vi "Enable Monitoring All Labels on Channel.vi"(8 "error in":errorcluster, 10 "channel number":u8, 11 "board handle":u8) -> (0 "error out":errorcluster, 2 "channel number out":u8, 3 "board handle out":u8)   [LabVIEW 2020, in "AIM ARINC 429 Hardware API.lvlib"]
uses:
  AIM ARINC 429 Hardware API.lvlib
  <instrlib>/AIM GmbH/_ARINC-429/subvi/Error Converter (ErrCode or Status).vi
  <instrlib>/AIM GmbH/_ARINC-429/subvi/Get Library Path.vi
  <instrlib>/AIM GmbH/_ARINC-429/VIs/Library/Api429Lib Error Desc Get.vi
  <instrlib>/AIM GmbH/_ARINC-429/subvi/Get Error Number Offset.vi
  <vilib>/Utility/error.llb/Error Cluster From Error Code.vi
  <instrlib>/AIM GmbH/_ARINC-429/AIM429LV.lvlib
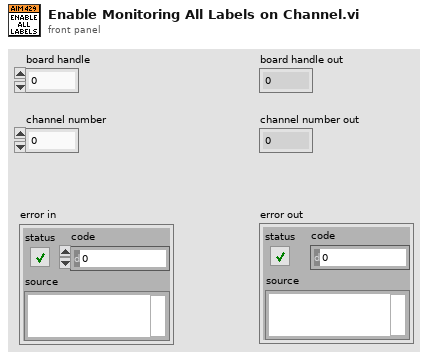
[diagram p1: front panel]
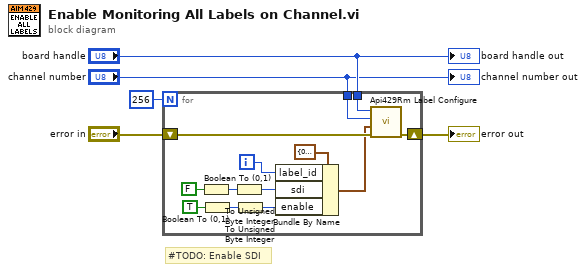
[diagram p0: block diagram]
diagram:
  # "#TODO: Enable SDI"
  n1 = for {
    N: 256 -> [_]
    tunnel: "board handle" -> [w18]
    tunnel: "channel number" -> [w17]
    shift-right: [w15] -> w2
    shift-left: "error in" -> [w16]
    i -> [w12]
    n2 = Boolean To (0,1)(Boolean=FALSE) -> (0, 1=w11:i16)
    n3 = Boolean To (0,1)(Boolean=TRUE) -> (0, 1=w7:i16)
    n4 = To Unsigned Byte Integer(number=w11) -> (unsigned 8bit integer=w9:u8)
    n5 = To Unsigned Byte Integer(number=w7) -> (unsigned 8bit integer=w6:u8)
    n6 = Bundle By Name(cluster=cluster{"label_id":u32, "sdi":u32, "enable":u8} {"label_id"=0, "sdi"=0, "enable"=0} ("label_config"), "label_id"=w12, "sdi"=w9, "enable"=w6) -> (w13:cluster{"label_id":u32, "sdi":u32, "enable":u8})
    n7 = call <instrlib>:"Api429Rm Label Configure.vi"("error in (no error)"=w16, "label_config"=w13, "b_Chn"=w17, "board_handle"=w18) -> ("error out"=w15:errorcluster)  [unwired: 7 in]
  }
  "error out" <- w2
  "board handle out" <- "board handle"
  "channel number out" <- "channel number"
